vi "备份参数.vi"() -> (0 "仪器公式":T1(array[cluster]), 1 "量程参数":T2(array[cluster]), 2 "试剂容量参数":T3, 3 "外设参数":T4, 5 "备份结果":string)   [LabVIEW 2016, in "斯坦道总磷.lvlib"]
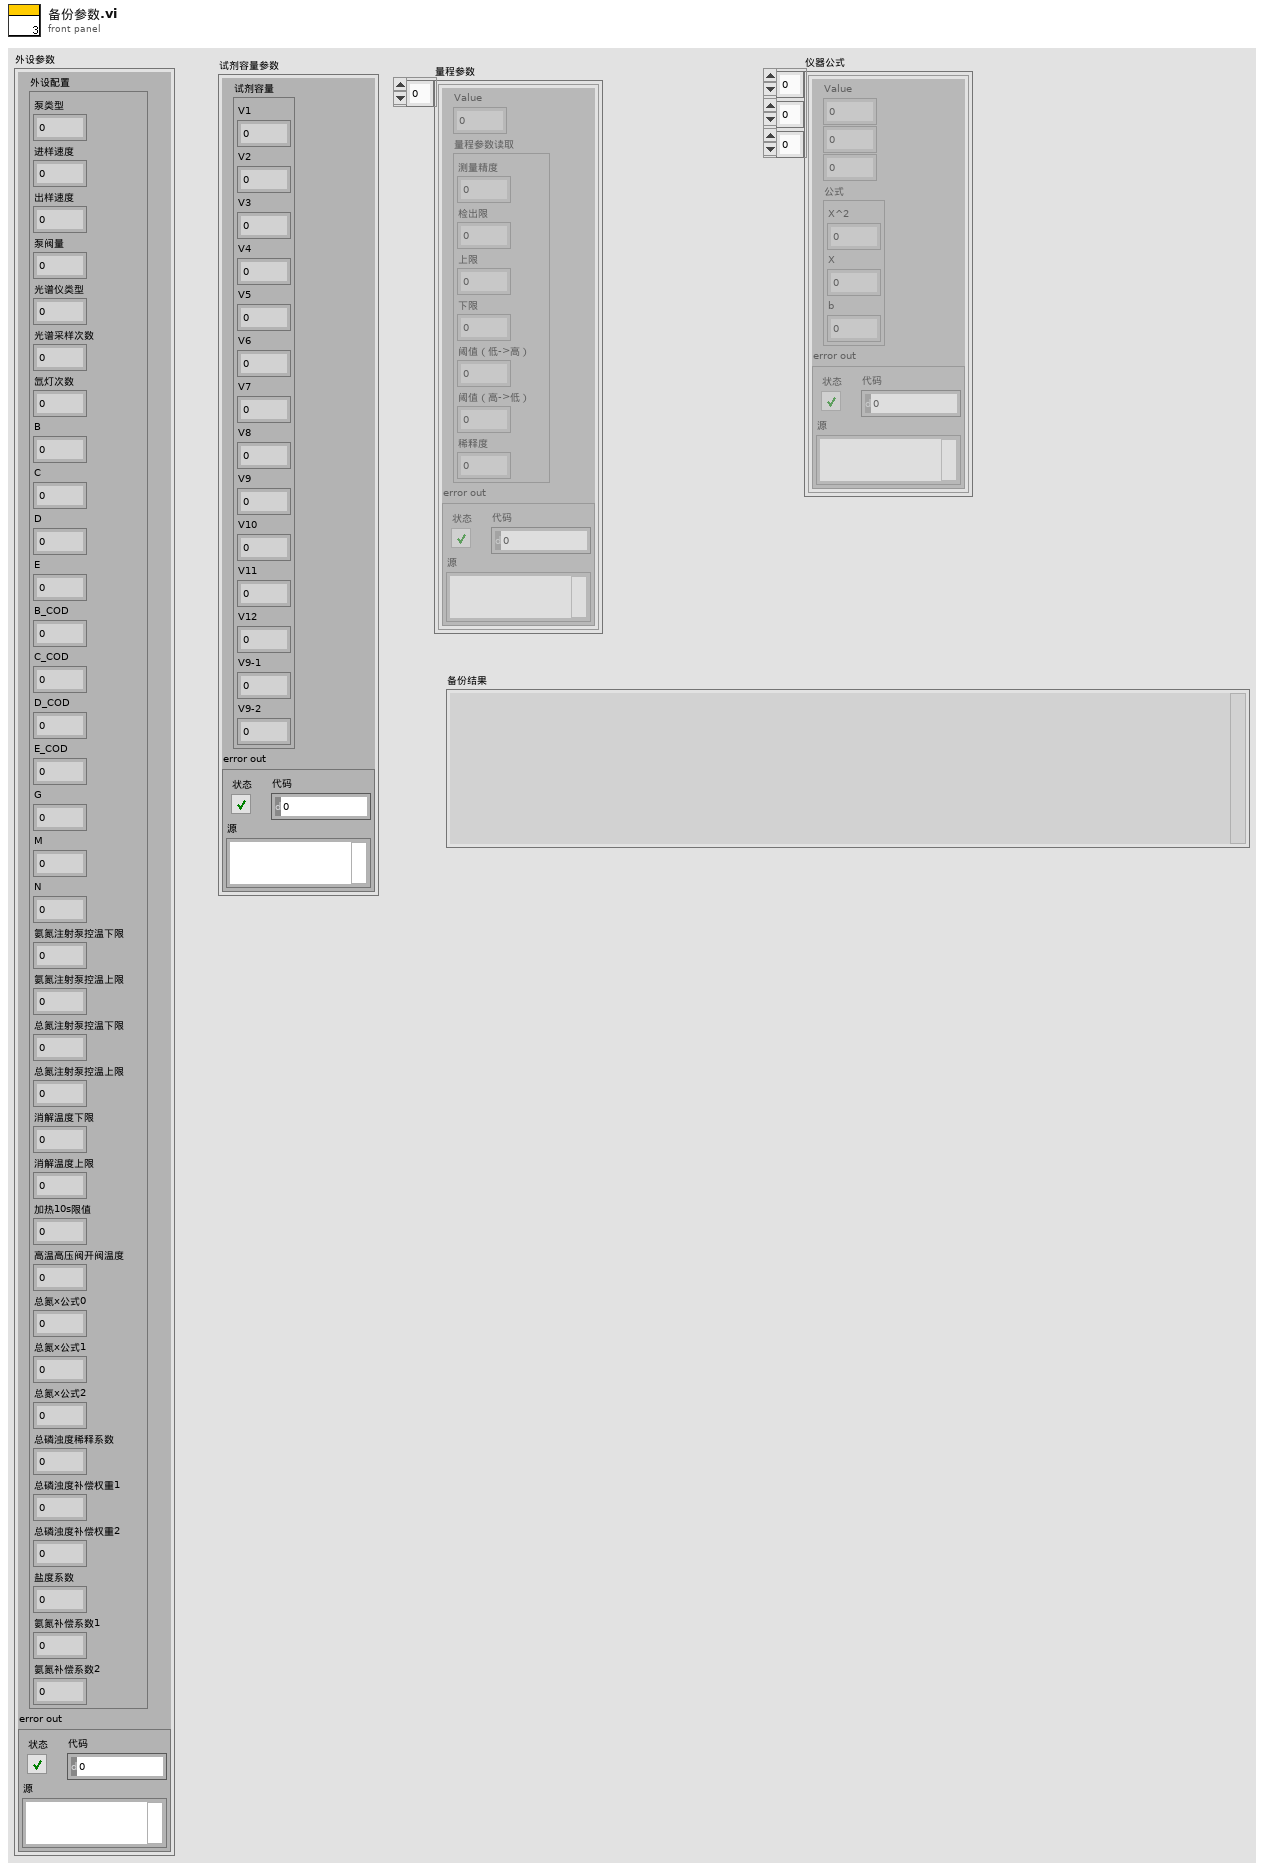
[diagram p1: front panel]
types:
  T1 = cluster{"Value":u16, i32, i32, "公式":cluster{"X^2":dbl, "X":dbl, "b":dbl}, "error out":errorcluster}[][][]
  T2 = cluster{"Value":u16, "量程参数读取":cluster{"测量精度":u16, "检出限":dbl, "上限":dbl, "下限":dbl, "阈值（低->高）":dbl, "阈值（高->低）":dbl, "稀释度":dbl}, "error out":errorcluster}[]
  T3 = cluster{"试剂容量":cluster{"V1":sgl, "V2":sgl, "V3":sgl, "V4":sgl, "V5":sgl, "V6":sgl, "V7":sgl, "V8":sgl, "V9":sgl, "V10":sgl, "V11":sgl, "V12":sgl, "V9-1":sgl, "V9-2":sgl}, "error out":errorcluster}
  T4 = cluster{"外设配置":cluster{"泵类型":u8, "进样速度":u32, "出样速度":u32, "泵阀量":u8, "光谱仪类型":u8, "光谱采样次数":u8, "氙灯次数":u8, "B":u16, "C":u16, "D":u16, "E":u16, "B_COD":u16, "C_COD":u16, "D_COD":u16, "E_COD":u16, "G":u16, "M":u16, "N":u16, "氨氮注射泵控温下限":sgl, "氨氮注射泵控温上限":sgl, "总氮注射泵控温下限":sgl, "总氮注射泵控温上限":sgl, "消解温度下限":sgl, "消解温度上限":sgl, "加热10s限值":sgl, "高温高压阀开阀温度":sgl, "总氮x公式0":u8, "总氮x公式1":sgl, "总氮x公式2":sgl, "总磷浊度稀释系数":sgl, "总磷浊度补偿权重1":sgl, "总磷浊度补偿权重2":sgl, "盐度系数":sgl, "氨氮补偿系数1":sgl, "氨氮补偿系数2":sgl}, "error out":errorcluster}
  T5 = enum16{"备份外设参数", "备份试剂容量参数", "备份量程参数", "备份仪器公式", "结束"}
  T6 = cluster{"泵类型":u8, "进样速度":u32, "出样速度":u32, "泵阀量":u8, "光谱仪类型":u8, "光谱采样次数":u8, "氙灯次数":u8, "B":u16, "C":u16, "D":u16, "E":u16, "B_COD":u16, "C_COD":u16, "D_COD":u16, "E_COD":u16, "G":u16, "M":u16, "N":u16, "氨氮注射泵控温下限":sgl, "氨氮注射泵控温上限":sgl, "总氮注射泵控温下限":sgl, "总氮注射泵控温上限":sgl, "消解温度下限":sgl, "消解温度上限":sgl, "加热10s限值":sgl, "高温高压阀开阀温度":sgl, "总氮x公式0":u8, "总氮x公式1":sgl, "总氮x公式2":sgl, "总磷浊度稀释系数":sgl, "总磷浊度补偿权重1":sgl, "总磷浊度补偿权重2":sgl, "盐度系数":sgl, "氨氮补偿系数1":sgl, "氨氮补偿系数2":sgl}
  T7 = cluster{"V1":sgl, "V2":sgl, "V3":sgl, "V4":sgl, "V5":sgl, "V6":sgl, "V7":sgl, "V8":sgl, "V9":sgl, "V10":sgl, "V11":sgl, "V12":sgl, "V9-1":sgl, "V9-2":sgl}
  T8 = cluster{"测量精度":u16, "检出限":dbl, "上限":dbl, "下限":dbl, "阈值（低->高）":dbl, "阈值（高->低）":dbl, "稀释度":dbl}
  T9 = cluster{"Value":u16, "量程参数读取":cluster{"测量精度":u16, "检出限":dbl, "上限":dbl, "下限":dbl, "阈值（低->高）":dbl, "阈值（高->低）":dbl, "稀释度":dbl}, "error out":errorcluster}
  T10 = cluster{"Value":u16, i32, i32, "公式":cluster{"X^2":dbl, "X":dbl, "b":dbl}, "error out":errorcluster}
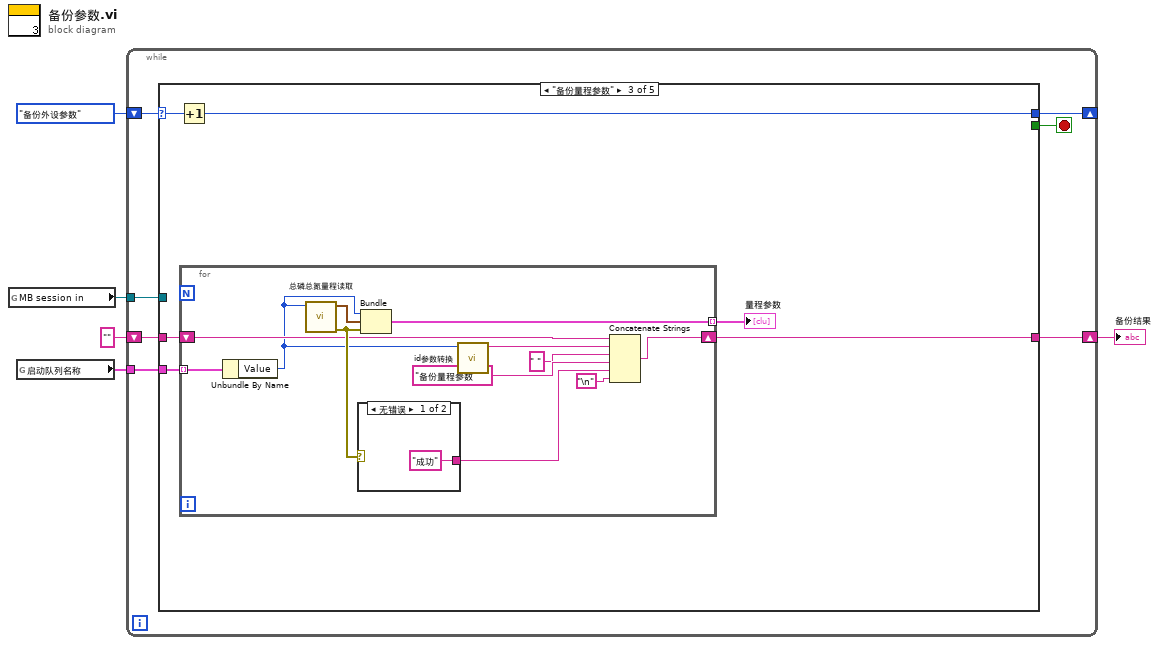
[diagram p0: block diagram]
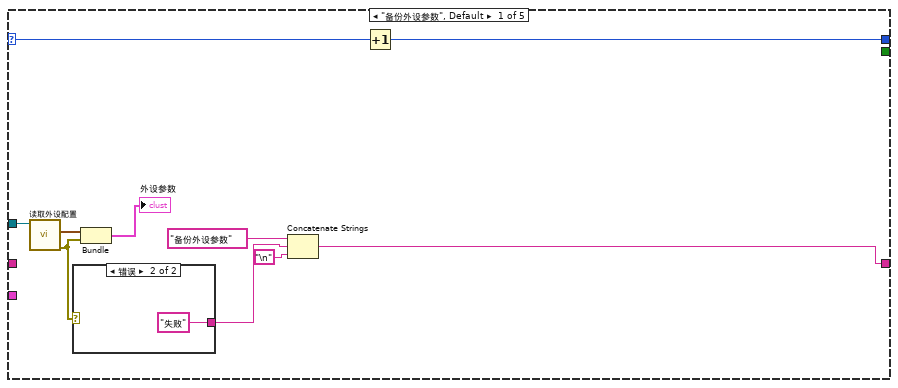
[diagram p2: hidden frame]
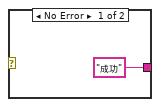
[diagram p3: hidden frame]
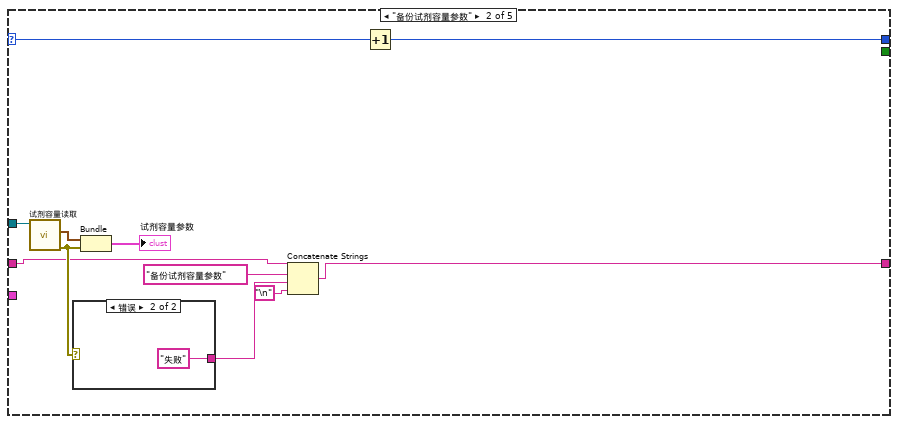
[diagram p4: hidden frame]
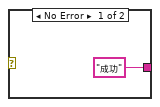
[diagram p5: hidden frame]
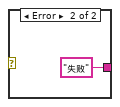
[diagram p6: hidden frame]
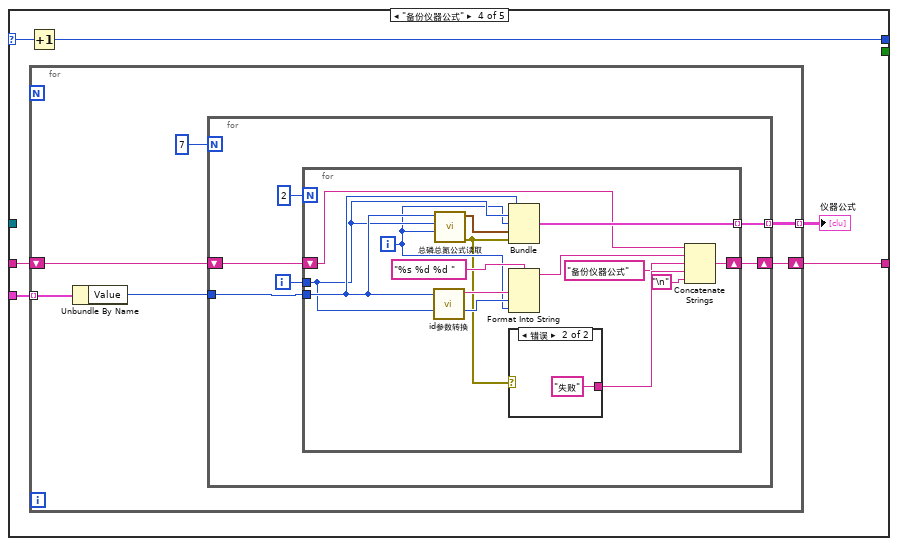
[diagram p7: hidden frame]
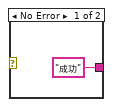
[diagram p8: hidden frame]
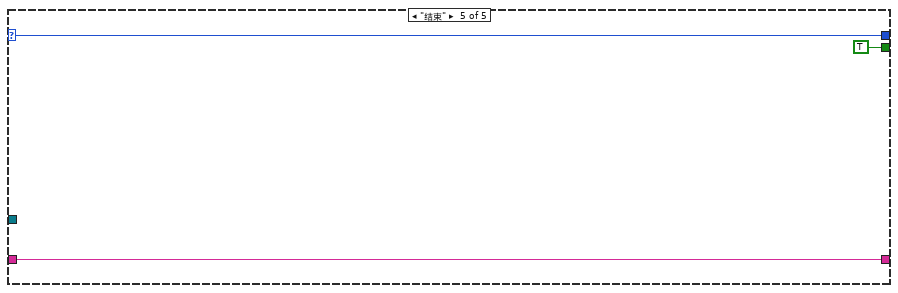
[diagram p9: hidden frame]
diagram:
  n1 = global read "VAR总磷总氮全局变量.vi" "MB session in"() -> (w4:refnum<class "MB_Master.lvclass">)
  n2 = global read "总磷总氮断电保存全局变量.vi" "启动队列名称"() -> (w2:cluster{"String":string, "Value":u16}[])
  n3 = while {
    shift-right: [w8] -> _
    shift-left: T5."备份外设参数" ("枚举") -> [w11]
    tunnel: w4 -> [w12]
    shift-right: [w9] -> w1
    shift-left: "" -> [w10]
    tunnel: w2 -> [w7]
    stop <- w6 stop-if-true
    n4 = case shown="\"备份量程参数\"" w11 {
      selector: w11 -> [w15 w27 w40 w60 w94]
      tunnel: w12 -> [w22 w35 _ _ _]
      tunnel: w10 -> [_ w29 w42 w62 w93]
      tunnel: [w17 w28 w41 w61 w93] -> w9
      tunnel: [w14 w26 w39 w59 w94] -> w8
      tunnel: w7 -> [_ _ w43 w63 _]
      tunnel: [_ _ _ _ TRUE] -> w6
      frame "备份外设参数", Default {
        n5 = call "读取外设配置.vi"("MB session in"=w22) -> ("error out"=w20:errorcluster, "外设配置"=w21:T6)  [unwired: 8 in, 1 out]
        n6 = case shown="错误" w20 {
          tunnel: ["成功" "失败"] -> w19
          frame No Error {
          }
          frame Error {
          }
        }
        n7 = Bundle("外设配置"=w21, "error out"=w20) -> (→"外设参数":T4)  [unwired: 1 in]
        n8 = Concatenate Strings("备份外设参数" ("字符串"), w19, "\n") -> (w17:string)
        n9 = Increment(x=w15) -> (x+1=w14:T5)
      }
      frame "备份试剂容量参数" {
        n10 = call "试剂容量读取.vi"("MB session in"=w35) -> ("error out"=w30:errorcluster, "试剂容量"=w34:T7)  [unwired: 8 in, 1 out]
        n11 = case shown="错误" w30 {
          tunnel: ["成功" "失败"] -> w33
          frame No Error {
          }
          frame Error {
          }
        }
        n12 = Bundle("试剂容量"=w34, "error out"=w30) -> (→"试剂容量参数":T3)  [unwired: 1 in]
        n13 = Concatenate Strings(w29, "备份试剂容量参数" ("字符串"), w33, "\n") -> (w28:string)
        n14 = Increment(x=w27) -> (x+1=w26:T5)
      }
      frame "备份量程参数" {
        n15 = Increment(x=w40) -> (x+1=w39:T5)
        n16 = for {
          tunnel: w43 -> [w55] mode=indexing
          tunnel: [w53] -> w38 mode=indexing
          shift-right: [w48] -> w41
          shift-left: w42 -> [w49]
          n17 = Unbundle By Name(w55) -> ("Value"=w47:u16)
          n18 = call "总磷总氮量程读取.vi"("测量参数"=w47) -> ("error out"=w50:errorcluster, "量程参数读取"=w54:T8)  [unwired: 9 in]
          n19 = case shown="无错误" w50 {
            tunnel: ["成功" "失败"] -> w52
            frame No Error {
            }
            frame Error {
            }
          }
          n20 = Bundle("Value"=w47, "量程参数读取"=w54, "error out"=w50) -> (w53:T9)  [unwired: 1 in]
          n21 = call "id参数转换.vi"("id"=w47) -> ("table输出"=w46:string)  [unwired: 9 in, 1 out]
          n22 = Concatenate Strings(w49, w46, " " ("字符串"), "备份量程参数" ("字符串"), w52, "\n") -> (w48:string)
        }
        "量程参数" <- w38
      }
      frame "备份仪器公式" {
        n23 = Increment(x=w60) -> (x+1=w59:T5)
        n24 = for {
          tunnel: w63 -> [w69] mode=indexing
          tunnel: [w66] -> w58 mode=indexing
          shift-right: [w64] -> w61
          shift-left: w62 -> [w65]
          n25 = Unbundle By Name(w69) -> ("Value"=w67:u16)
          n26 = for {
            N: 7 -> [_]
            tunnel: w67 -> [w75]
            tunnel: [w72] -> w66 mode=indexing
            shift-right: [w71] -> w64
            shift-left: w65 -> [w70]
            i -> [w74]
            n27 = for {
              N: 2 -> [_]
              tunnel: w75 -> [w83]
              tunnel: w74 -> [w80]
              tunnel: [w88] -> w72 mode=indexing
              shift-right: [w85] -> w71
              shift-left: w70 -> [w84]
              i -> [w79]
              n28 = call "id参数转换.vi"("id"=w83) -> ("table输出"=w81:string)  [unwired: 9 in, 1 out]
              n29 = call "总磷总氮公式读取.vi"("量程"=w79, "测量模式"=w80, "测量参数"=w83) -> ("error out"=w77:errorcluster, "公式"=w89:cluster{"X^2":dbl, "X":dbl, "b":dbl})  [unwired: 7 in]
              n30 = Bundle("Value"=w83, w80, w79, "公式"=w89, "error out"=w77) -> (w88:T10)  [unwired: 1 in]
              n31 = Format Into String(format string="%s %d %d " ("格式字符串"), w81, w80, w79) -> (resulting string=w78:string)  [unwired: 2 in, 1 out]
              n32 = case shown="错误" w77 {
                tunnel: ["成功" "失败"] -> w87
                frame No Error {
                }
                frame Error {
                }
              }
              n33 = Concatenate Strings(w84, w78, "备份仪器公式" ("字符串"), w87, "\n") -> (w85:string)
            }
          }
        }
        "仪器公式" <- w58
      }
      frame "结束" {
      }
    }
  }
  "备份结果" <- w1
